vi "Sensitivity limit (SubVI).vi"(8 "error in (no error)":errorcluster, 11 "Instrument parameters in":T1) -> (0 "error out":errorcluster, 2 "Sensitivity out":dbl, 3 "Instrument parameters out":T1)   [LabVIEW 2016, in "MyLockIn.lvlib"]
uses:
  MyLockIn.lvlib
  TYPE DEFS/S2DS_Instrument parameters.ctl
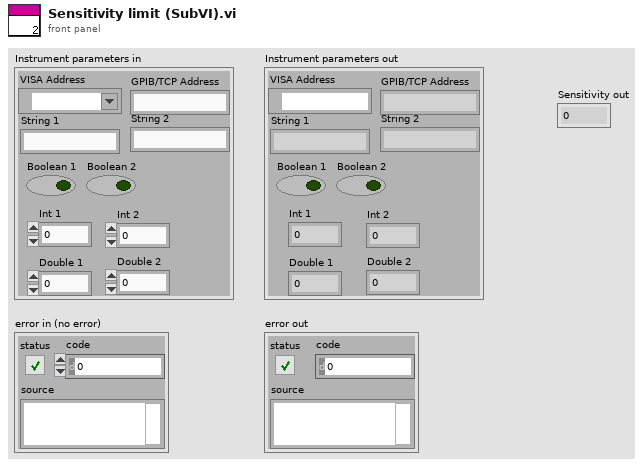
[diagram p1: front panel]
types:
  T1 = typedef "S2DS_Instrument parameters.ctl" = cluster{"VISA Address":refnum<visa-resource-name>, "GPIB/TCP Address":string, "String 1":string, "String 2":string, "Boolean 1":bool, "Boolean 2":bool, "Int 1":i32, "Int 2":i32, "Double 1":dbl, "Double 2":dbl}
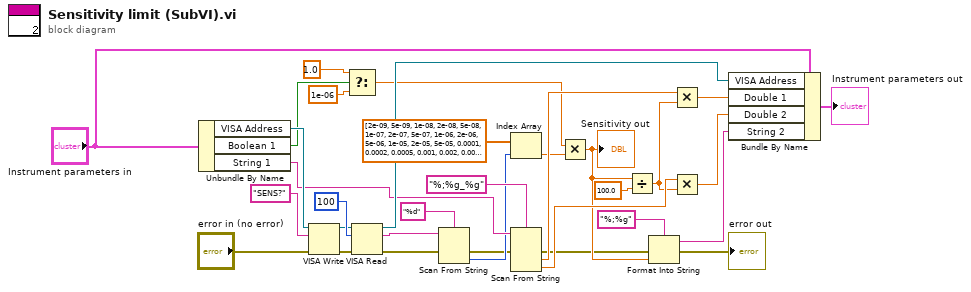
[diagram p0: block diagram]
diagram:
  n1 = Unbundle By Name("Instrument parameters in") -> ("VISA Address"=w31:refnum<visa-resource-name>, "Boolean 1"=w19:bool, "String 1"=w30:string)
  n2 = VISA Write(VISA resource name=w31, write buffer="SENS?", error in (no error)="error in (no error)") -> (VISA resource name out=w10:refnum<visa-resource-name>, error out=w11:errorcluster)  [unwired: 1 out]
  n3 = Select(t=1.0, s=w19, f=1e-06) -> (s? t:f=w22:dbl)
  n4 = VISA Read(VISA resource name=w10, byte count=u32 100, error in (no error)=w11) -> (VISA resource name out=w32:refnum<visa-resource-name>, read buffer=w14:string, error out=w16:errorcluster)  [unwired: 1 out]
  n5 = Scan From String(format string="%d", input string=w14, error in=w16) -> (error out=w3:errorcluster, output 1=w17:i32)  [unwired: 2 in, 2 out]
  n6 = Index Array(array=dbl[] [2e-09, 5e-09, 1e-08, 2e-08, 5e-08, 1e-07, 2e-07, 5e-07, 1e-06, 2e-06, 5e-06, 1e-05, 2e-05, 5e-05, 0.0001, 0.0002, 0.0005, 0.001, 0.002, 0.005, 0.01, 0.02, 0.05, 0.1, 0.2, 0.5], index=w17) -> (element=w23:dbl)
  n7 = Scan From String(format string="%;%g_%g", input string=w30, error in=w3) -> (error out=w2:errorcluster, output 1=w25:dbl, output 2=w26:dbl)  [unwired: 3 in, 2 out]
  n8 = Multiply(x=w22, y=w23) -> (x*y=w6:dbl)
  "Sensitivity out" <- w6
  n9 = Divide(x=w6, y=100.0) -> (x/y=w7:dbl)
  n10 = Format Into String(format string="%;%g", error in=w2, w6) -> (resulting string=w4:string, error out=→"error out":errorcluster)  [unwired: 1 in]
  n11 = Multiply(x=w25, y=w7) -> (x*y=w28:dbl)
  n12 = Multiply(x=w26, y=w7) -> (x*y=w29:dbl)
  n13 = Bundle By Name(cluster="Instrument parameters in", "VISA Address"=w32, "Double 1"=w28, "Double 2"=w29, "String 2"=w4) -> (→"Instrument parameters out":T1)
